vi "CSM - Filter By Option.vi"(1 "Option":T1(ring), 5 "State (S) In (\"\")":string, 7 "Filter String":string) -> (6 "States Out":string)   [LabVIEW 2017]
doc: "Filter messages sent to non-existing modules.\nThis VI uses CSM - List Modules.vi to get all active CSM modules and then filters out messages sent to non-existing modules.\n\n-- <b>Controls</b> --\n- <b>States</b>: Input message string\n\n-- <b>Indicators</b> --\n- <b>Filtered States</b>: Filtered message string"
uses:
  user.lib/_NEVSTOP/Communicable State Machine(CSM)/Communicable State Machine.lvlib
  user.lib/_NEVSTOP/Communicable State Machine(CSM)/_Shared/CSM Shared.lvlib
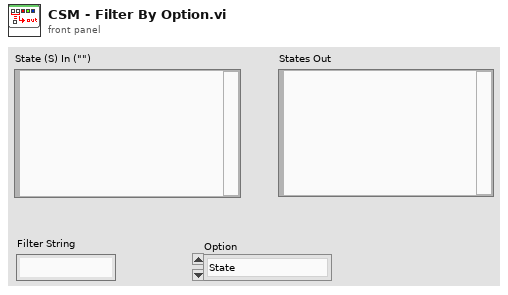
[diagram p1: front panel]
types:
  T1 = enum16{"State", "State+Arg", "Target", "Message", "NoComments", "RawString"}
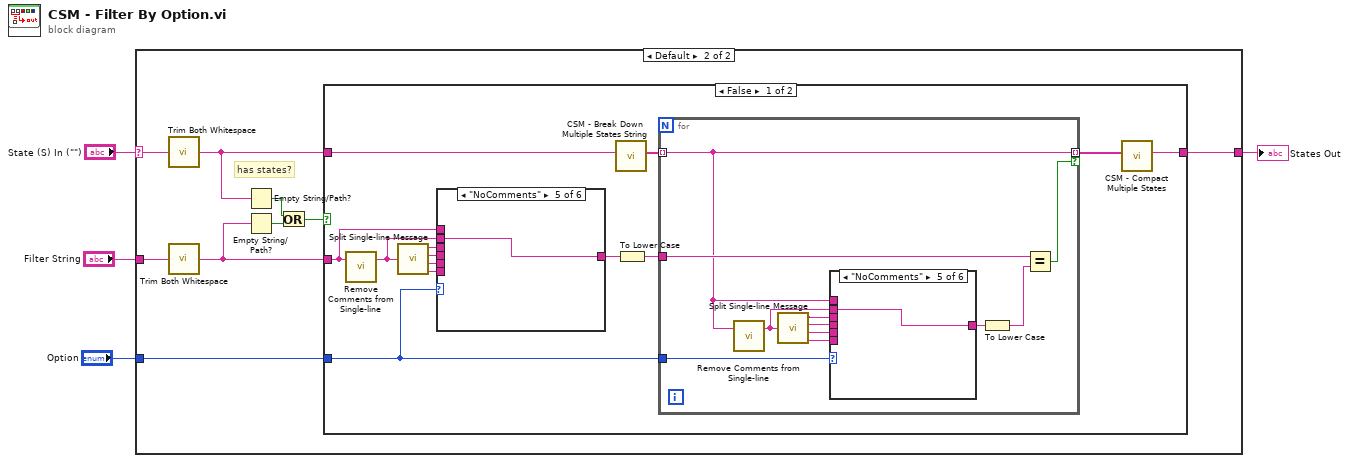
[diagram p0: block diagram]
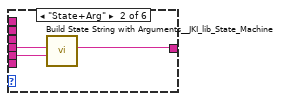
[diagram p4: hidden frame]
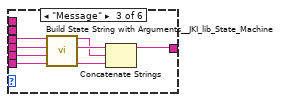
[diagram p5: hidden frame]
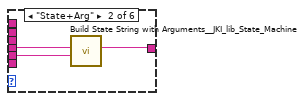
[diagram p9: hidden frame]
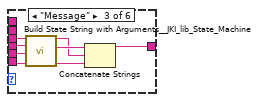
[diagram p10: hidden frame]
diagram:
  n1 = case shown="Default" "State (S) In (\"\")" {
    selector: "State (S) In (\"\")" -> [_ w11]
    tunnel: [_ w13] -> w3
    tunnel: "Filter String" -> [_ w9]
    tunnel: "Option" -> [_ w10]
    frame "" {
    }
    frame Default {
      # "has states?"
      n2 = call "Trim Both Whitespace.vi"("string"=w11) -> ("trimmed string"=w12:string)  [unwired: 1 in]
      n3 = call "Trim Both Whitespace.vi"("string"=w9) -> ("trimmed string"=w5:string)  [unwired: 1 in]
      n4 = Empty String/Path?(string/path=w12) -> (empty?=w7:bool)
      n5 = Empty String/Path?(string/path=w5) -> (empty?=w8:bool)
      n6 = Or(x=w7, y=w8) -> (x .or. y?=w6:bool)
      n7 = case shown="False" w6 {
        tunnel: w12 -> [w26 w64]
        tunnel: [w25 w64] -> w13
        tunnel: w10 -> [w19 _]
        tunnel: w5 -> [w14 _]
        frame False {
          n8 = call "Remove Comments from Single-line.vi"("single-line text"=w14) -> ("single-line text without comments"=w16:string)  [unwired: 2 in]
          n9 = call "Split Single-line Message.vi"("single-line text"=w16) -> ("operator"=w15:string, "state"=w22:string, "args"=w21:string, "source/target"=w17:string)  [unwired: 6 in]
          n10 = case shown="\"NoComments\"" w19 {
            tunnel: w22 -> [w27 w29 w35 _ _ _]
            tunnel: w21 -> [_ w30 w36 _ _ _]
            tunnel: [w27 w28 w33 w37 w38 w39] -> w20
            tunnel: w17 -> [_ _ w32 w37 _ _]
            tunnel: w16 -> [_ _ _ _ w38 _]
            tunnel: w15 -> [_ _ w31 _ _ _]
            tunnel: w14 -> [_ _ _ _ _ w39]
            frame "State", Default {
            }
            frame "State+Arg" {
              n11 = call <vilib>:"Build State String with Arguments__JKI_lib_State_Machine.vi"("Arguments (\"\")"=w30, "State"=w29) -> ("State with Arguments"=w28:string)  [unwired: 4 in]
            }
            frame "Message" {
              n12 = call <vilib>:"Build State String with Arguments__JKI_lib_State_Machine.vi"("Arguments (\"\")"=w36, "State"=w35) -> ("State with Arguments"=w34:string)  [unwired: 4 in]
              n13 = Concatenate Strings(w34, w31, w32) -> (w33:string)
            }
            frame "Target" {
            }
            frame "NoComments" {
            }
            frame "RawString" {
            }
          }
          n14 = call "CSM - Break Down Multiple States String.vi"("States"=w26) -> ("Multiple States"=w24:string[])  [unwired: 10 in]
          n15 = To Lower Case(string=w20) -> (all lower case string=w18:string)
          n16 = for {
            tunnel: w24 -> [w40] mode=indexing
            tunnel: [w40] -> w23 mode=indexing if=w47
            tunnel: w18 -> [w45]
            tunnel: w19 -> [w48]
            n17 = call "Remove Comments from Single-line.vi"("single-line text"=w40) -> ("single-line text without comments"=w42:string)  [unwired: 2 in]
            n18 = call "Split Single-line Message.vi"("single-line text"=w42) -> ("operator"=w41:string, "state"=w50:string, "args"=w49:string, "source/target"=w43:string)  [unwired: 6 in]
            n19 = case shown="\"NoComments\"" w48 {
              tunnel: w50 -> [w51 w53 w59 _ _ _]
              tunnel: w49 -> [_ w54 w58 _ _ _]
              tunnel: [w51 w52 w55 w61 w62 w63] -> w46
              tunnel: w43 -> [_ _ w57 w61 _ _]
              tunnel: w42 -> [_ _ _ _ w62 _]
              tunnel: w41 -> [_ _ w56 _ _ _]
              tunnel: w40 -> [_ _ _ _ _ w63]
              frame "State", Default {
              }
              frame "State+Arg" {
                n20 = call <vilib>:"Build State String with Arguments__JKI_lib_State_Machine.vi"("Arguments (\"\")"=w54, "State"=w53) -> ("State with Arguments"=w52:string)  [unwired: 4 in]
              }
              frame "Message" {
                n21 = call <vilib>:"Build State String with Arguments__JKI_lib_State_Machine.vi"("Arguments (\"\")"=w58, "State"=w59) -> ("State with Arguments"=w60:string)  [unwired: 4 in]
                n22 = Concatenate Strings(w60, w56, w57) -> (w55:string)
              }
              frame "Target" {
              }
              frame "NoComments" {
              }
              frame "RawString" {
              }
            }
            n23 = To Lower Case(string=w46) -> (all lower case string=w44:string)
            n24 = Equal?(x=w45, y=w44) -> (x = y?=w47:bool)
          }
          n25 = call "CSM - Compact Multiple States.vi"("Multiple States"=w23) -> ("States"=w25:string)  [unwired: 9 in]
        }
        frame True {
        }
      }
    }
  }
  "States Out" <- w3
